vi "flt_sos8xblock.vi"(7 "sosBypass":bool[](array[boolean])=[FALSE, FALSE, FALSE, FALSE, FALSE, FALSE, FALSE, FALSE], 8 "input valid":bool, 9 "b":fxp<+/-,24,8>[](array[numeric])=[0.0, 0.0, 0.0, 0.0, 0.0, 0.0, 0.0, 0.0, 0.0, 0.0, 0.0, 0.0, 0.0, 0.0, 0.0, 0.0, 0.0, 0.0, 0.0, 0.0, 0.0, 0.0, 0.0, 0.0], 10 "anot":fxp<+/-,24,8>[](array[numeric])=[0.0, 0.0, 0.0, 0.0, 0.0, 0.0, 0.0, 0.0, 0.0, 0.0, 0.0, 0.0, 0.0, 0.0, 0.0, 0.0], 11 "input":fxp<+/-,28,1>) -> (0 "ready for input":bool, 1 "output valid":bool, 3 "output":fxp<+/-,20,2>)   [LabVIEW 2016]
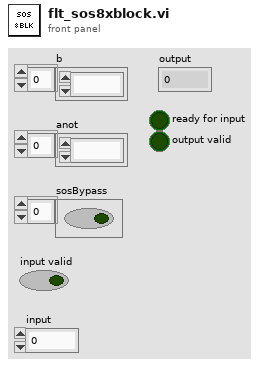
[diagram p1: front panel]
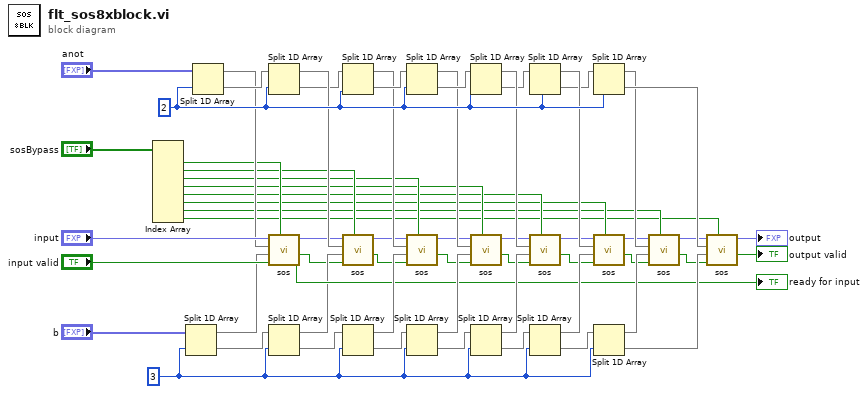
[diagram p0: block diagram]
diagram:
  w48 = 3 ("length")
  w60 = 2 ("length")
  n1 = Index Array(array="sosBypass") -> (element #1=w8:bool, element #2=w7:bool, element #3=w6:bool, element #4=w5:bool, element #5=w4:bool, element #6=w3:bool, element #7=w2:bool, element #8=w1:bool)  [unwired: 8 in]
  n2 = Split 1D Array(array="b", index=w48) -> (first subarray=w27:fxp<+/-,24,8>[], second subarray=w24:fxp<+/-,24,8>[])
  n3 = Split 1D Array(array="anot", index=w60) -> (first subarray=w18:fxp<+/-,24,8>[], second subarray=w19:fxp<+/-,24,8>[])
  n4 = Split 1D Array(array=w19, index=w60) -> (first subarray=w21:fxp<+/-,24,8>[], second subarray=w20:fxp<+/-,24,8>[])
  n5 = call "sos.vi"("bypass"=w8, "input valid"="input valid", "b"=w27, "anot"=w18, "input"="input") -> ("ready for input"=→"ready for input":bool, "output valid"=w16:bool, "output"=w13:fxp<+/-,26,9>)  [unwired: 4 in]
  n6 = Split 1D Array(array=w24, index=w48) -> (first subarray=w26:fxp<+/-,24,8>[], second subarray=w25:fxp<+/-,24,8>[])
  n7 = Split 1D Array(array=w20, index=w60) -> (first subarray=w22:fxp<+/-,24,8>[], second subarray=w50:fxp<+/-,24,8>[])
  n8 = call "sos.vi"("bypass"=w7, "input valid"=w16, "b"=w26, "anot"=w21, "input"=w13) -> ("output valid"=w15:bool, "output"=w12:fxp<+/-,26,9>)  [unwired: 4 in, 1 out]
  n9 = Split 1D Array(array=w25, index=w48) -> (first subarray=w44:fxp<+/-,24,8>[], second subarray=w40:fxp<+/-,24,8>[])
  n10 = Split 1D Array(array=w50, index=w60) -> (first subarray=w49:fxp<+/-,24,8>[], second subarray=w51:fxp<+/-,24,8>[])
  n11 = call "sos.vi"("bypass"=w6, "input valid"=w15, "b"=w44, "anot"=w22, "input"=w12) -> ("output valid"=w14:bool, "output"=w11:fxp<+/-,26,9>)  [unwired: 4 in, 1 out]
  n12 = Split 1D Array(array=w40, index=w48) -> (first subarray=w45:fxp<+/-,24,8>[], second subarray=w41:fxp<+/-,24,8>[])
  n13 = Split 1D Array(array=w51, index=w60) -> (first subarray=w56:fxp<+/-,24,8>[], second subarray=w52:fxp<+/-,24,8>[])
  n14 = call "sos.vi"("bypass"=w5, "input valid"=w14, "b"=w45, "anot"=w49, "input"=w11) -> ("output valid"=w34:bool, "output"=w38:fxp<+/-,26,9>)  [unwired: 4 in, 1 out]
  n15 = Split 1D Array(array=w41, index=w48) -> (first subarray=w46:fxp<+/-,24,8>[], second subarray=w42:fxp<+/-,24,8>[])
  n16 = Split 1D Array(array=w52, index=w60) -> (first subarray=w57:fxp<+/-,24,8>[], second subarray=w53:fxp<+/-,24,8>[])
  n17 = call "sos.vi"("bypass"=w4, "input valid"=w34, "b"=w46, "anot"=w56, "input"=w38) -> ("output valid"=w35:bool, "output"=w31:fxp<+/-,26,9>)  [unwired: 4 in, 1 out]
  n18 = Split 1D Array(array=w42, index=w48) -> (first subarray=w47:fxp<+/-,24,8>[], second subarray=w43:fxp<+/-,24,8>[])
  n19 = Split 1D Array(array=w53, index=w60) -> (first subarray=w58:fxp<+/-,24,8>[], second subarray=w59:fxp<+/-,24,8>[])
  n20 = call "sos.vi"("bypass"=w3, "input valid"=w35, "b"=w47, "anot"=w57, "input"=w31) -> ("output valid"=w36:bool, "output"=w32:fxp<+/-,26,9>)  [unwired: 4 in, 1 out]
  n21 = Split 1D Array(array=w43, index=w48) -> (first subarray=w54:fxp<+/-,24,8>[], second subarray=w55:fxp<+/-,24,8>[])
  n22 = call "sos.vi"("bypass"=w2, "input valid"=w36, "b"=w54, "anot"=w58, "input"=w32) -> ("output valid"=w37:bool, "output"=w33:fxp<+/-,26,9>)  [unwired: 4 in, 1 out]
  n23 = call "sos.vi"("bypass"=w1, "input valid"=w37, "b"=w55, "anot"=w59, "input"=w33) -> ("output valid"=→"output valid":bool, "output"=→"output":fxp<+/-,26,9>)  [unwired: 4 in, 1 out]
